vi "Temp and Luz.vi"(8 "Error In":errorcluster, 9 "Pin LM35":u8, 10 "Pin Fotoresistencia":u8, 11 "Serial Port":refnum<visa-resource-name>="N/A") -> (0 "Error Out":errorcluster, 2 "Temp. Ambiental.":dbl, 3 "LUZ":dbl)   [LabVIEW 2013]
uses:
  <vilib>/MakerHub/LINX/Private/Type Defs/User Platform.ctl
  <vilib>/MakerHub/LINX/Private/Type Defs/Interface.ctl
  <vilib>/MakerHub/LINX/Public/Sensors/Temperature/TMP3x/TMP35.vi
  <vilib>/MakerHub/LINX/LMH-LINX.lvlib
  <vilib>/MakerHub/LINX/Public/Sensors/Temperature/TMP3x/TMP3x.lvlib
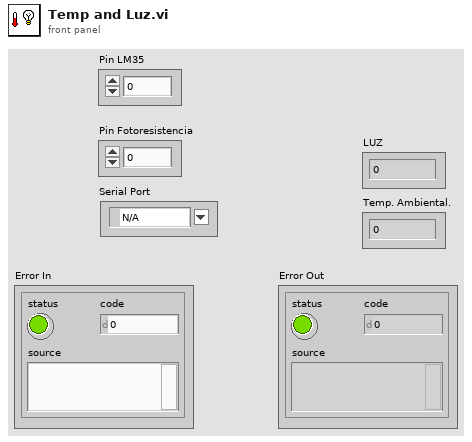
[diagram p1: front panel]
types:
  T1 = typedef "LMH-LINX.lvlib/Interface.ctl" = enum16{"Serial", "TCP"}
  T2 = typedef "LMH-LINX.lvlib/User Platform.ctl" = enum16{"Default", "LINX", "myRIO"}
  T3 = typedef "LMH-LINX.lvlib/LINX Ref.ctl" = cluster{"Platform":T4, "Interface":T1, "LINX Device Config":T5}
  T4 = typedef "LMH-LINX.lvlib/Platform.ctl" = enum16{"LINX", "myRIO"}
  T5 = typedef "LMH-LINX.lvlib/Device.lvlib/LINX Device Config.ctl" = cluster{"Interface":T1, "COM Port":refnum<visa-resource-name>, "TCP Configuration":T6, "Device Family":u8, "Device ID":u8, "Device Name":string, "TCP Ref":refnum<k5>, "Channels":T7}
  T6 = typedef "LMH-LINX.lvlib/Device.lvlib/TCP Config.ctl" = cluster{"IP Address":string, "Port":u16}
  T7 = typedef "LMH-LINX.lvlib/Channels.ctl" = cluster{"DI":u8[], "DO":u8[], "AI":u8[], "AO":u8[], "PWM":u8[], "QE":u8[], "UART":u8[], "I2C 2":u8[], "SPI":u8[], "CAN":u8[], "Servo":u8[], "AI Ref (V)":dbl, "AO Ref (V)":dbl, "AO Resolution (Bits)":u8}
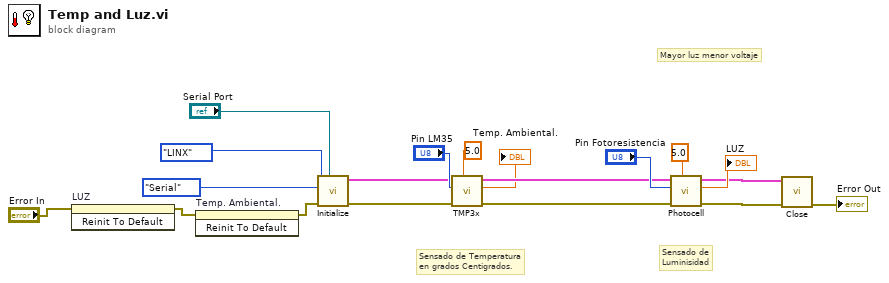
[diagram p0: block diagram]
diagram:
  # "Mayor luz menor voltaje"
  # "Sensado de\nLuminisidad"
  # "Sensado de Temperatura\nen grados Centigrados."
  n1 = invoke on="LUZ" class="DigNum (strict)" method="Reinit To Default"(error in="Error In") -> (error out=w2:errorcluster)  [unwired: 2 in, 2 out]
  n2 = invoke on="Temp. Ambiental." class="DigNum (strict)" method="Reinit To Default"(error in=w2) -> (error out=w1:errorcluster)  [unwired: 2 in, 2 out]
  n3 = call <vilib>:"Initialize.vi"("Serial Port"="Serial Port", "Error In"=w1, "Interface"=Interface."Serial", "Platform"=User_Platform."LINX") -> ("Error Out"=w6:errorcluster, "LINX Ref"=w7:T3)  [unwired: 5 in, 1 out]
  n4 = call-poly <vilib>:"TMP3x.vi"("Analog Ref Override"=5.0, "Error In"=w6, "Analog Channel"="Pin LM35", "LINX Resource"=w7) -> ("Error Out"=w10:errorcluster, "Temp C"=→"Temp. Ambiental.":dbl, "LINX Resource"=w9:T3)  [unwired: 5 in]
  n5 = call <vilib>:"Photocell.vi"("Analog Ref Override"=5.0, "Error In"=w10, "AI Channel"="Pin Fotoresistencia", "LINX Resource"=w9) -> ("Error Out"=w4:errorcluster, "Value (0-100)"=→"LUZ":dbl, "LINX Resource"=w5:T3)  [unwired: 5 in]
  n6 = call <vilib>:"Close.vi"("Error In"=w4, "LINX Resource"=w5) -> ("Error Out"=→"Error Out":errorcluster)  [unwired: 8 in, 1 out]
